vi "Activity_1(P1).vi"() -> ()   [LabVIEW 2019]
panel:
  out "Temp Out *C":dbl(slide) scale=-100.0..100.0
  out "Temp Out *F":dbl(slide) scale=-100.0..100.0
  in  "Temp in *C":dbl
  in  "Temp in *F":dbl
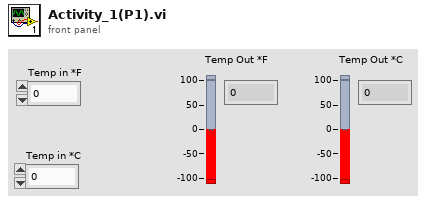
[diagram p1: front panel]
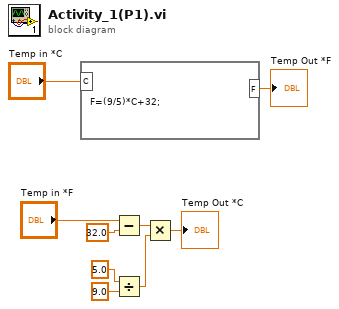
[diagram p0: block diagram]
diagram:
  n1 = formula code="F=(9/5)*C+32;"("C"="Temp in *C") -> ("F"=→"Temp Out *F":dbl)
  n2 = Subtract(x="Temp in *F", y=32.0) -> (x-y=w7:dbl)
  n3 = Divide(x=5.0, y=9.0) -> (x/y=w4:dbl)
  n4 = Multiply(x=w7, y=w4) -> (x*y=→"Temp Out *C":dbl)
